vi "Operator Login Dialog.vi"(8 "error in (no error)":errorcluster, 9 "contextType":i32(ring) items=["Machine", "Domain", "ApplicationDirectory"]) -> (0 "error out":errorcluster, 1 "Groups":string[](array[string]), 2 "Operator Name":string, 3 "Logged In?":bool)   [LabVIEW 2020, in "Common Dialogs.lvlib"]
doc: "Use this template to create a dialog box with event handling."
uses:
  Common Dialogs.lvlib
  System.DirectoryServices.AccountManagement
panel:
  in  "Password":string
  in  "Operator Name":string
  in  "Cancel":bool
  in  "Login":bool
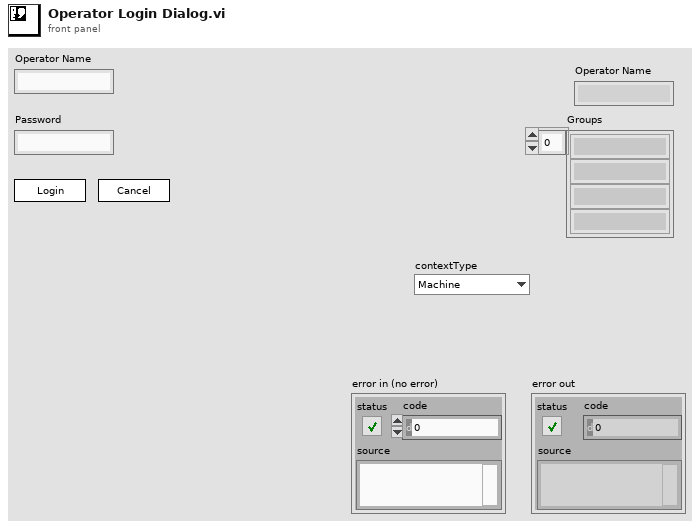
[diagram p1: front panel]
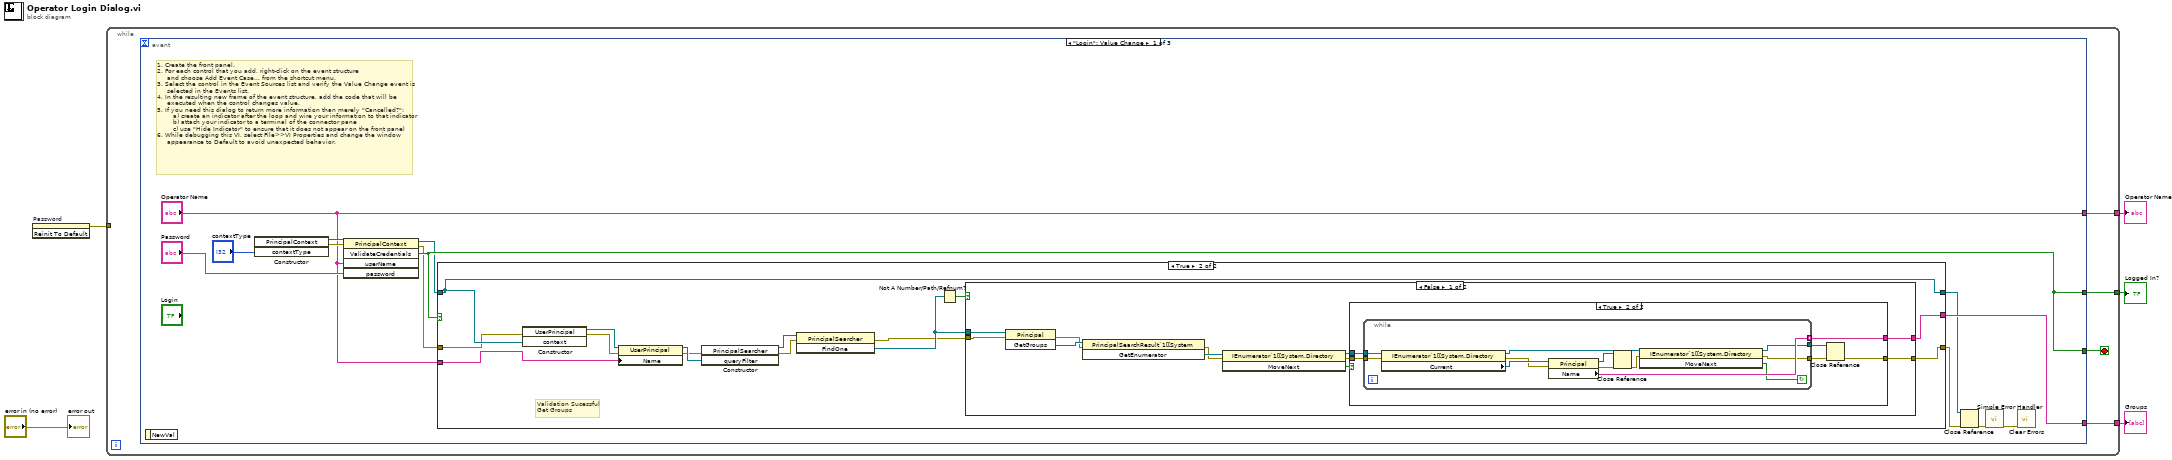
[diagram p0: block diagram]
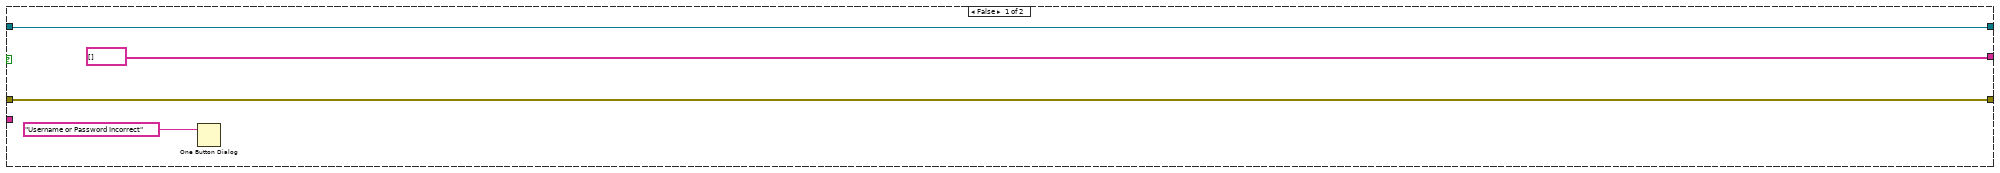
[diagram p2: hidden frame]
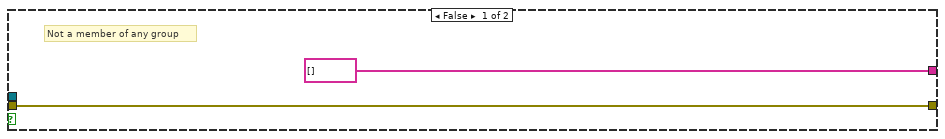
[diagram p3: hidden frame]
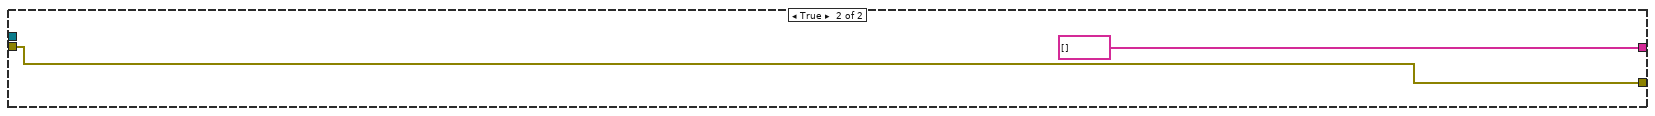
[diagram p4: hidden frame]
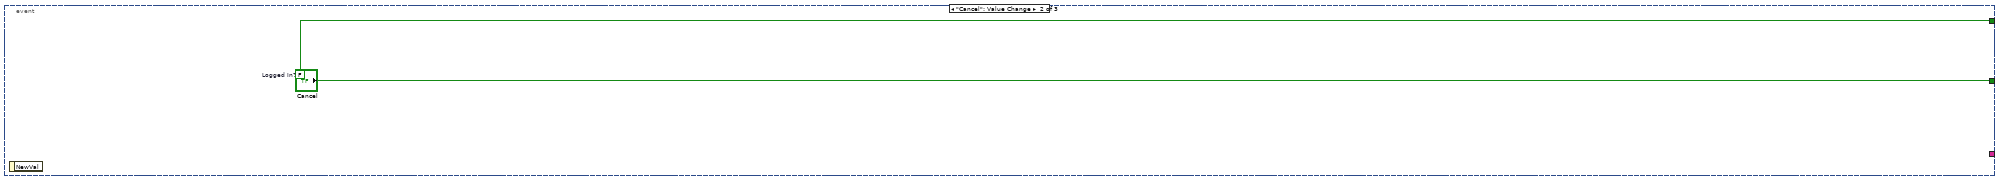
[diagram p5: hidden frame]
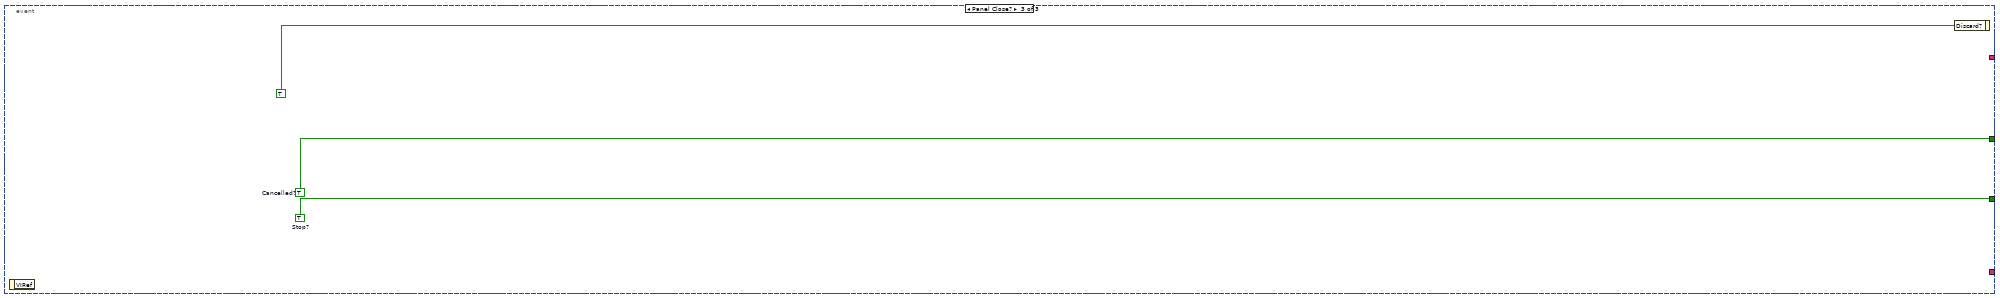
[diagram p6: hidden frame]
diagram:
  n1 = invoke on="Password" class="Str" method="Reinit To Default"() -> (error out=w2:errorcluster)  [unwired: 3 in, 2 out]
  n2 = while {
    tunnel: [w8] -> w5
    tunnel: [w7] -> w4
    tunnel: [w6] -> w3
    tunnel: w2 -> [_]
    stop <- w9 stop-if-true
    n3 = event shown="[0] \"Login\": Value Change" {
      selector: _ -> [_ _ _]
      dyn-events: _ -> [_ _ _]
      timeout: _ -> [_ _ _]
      tunnel: [w18 "Cancel" w77] -> w9
      tunnel: [w18 w75 w76] -> w8
      tunnel: ["Operator Name" _ _] -> w7
      tunnel: [w15 _ _] -> w6
      event "Login": Value Change {
        # "1. Create the front panel.\n2. For each control that you add, right-click on the event structure \n     and choose Add Event Case... from the shortcut menu.\n3. Select the control in the Event Sources list and verify the Value Change event is \n     selected in the Events list.\n4. In the resulting new frame of the event structure, add the code that will be \n     executed when the control changes value.\n5. If you need this dialog to return more information than merely \"Cancelled?\":\n        a) create an indicator after the loop and wire your information to that indicator\n        b) attach your indicator to a terminal of the connector pane\n        c) use \"Hide Indicator\" to ensure that it does not appear on the front panel\n6. While debugging this VI, select File>>VI Properties and change the window \n     appearance to Default to avoid unexpected behavior."
        n4 = event-data() -> ()  [unwired: 1 in, 1 out]
        n5 = constructor class="PrincipalContext"("contextType"="contextType") -> (reference out=w20:refnum<k24>, error out=w21:errorcluster)  [unwired: 3 in, 2 out]
        n6 = invoke class="PrincipalContext" method="ValidateCredentials"(reference=w20, error in=w21, "userName"="Operator Name", "password"="Password") -> (reference out=w14:refnum<k24>, error out=w13:errorcluster, "ValidateCredentials"=w18:bool)  [unwired: 1 in, 2 out]
        n7 = case shown="True" w18 {
          tunnel: [string[] [] ("Groups") w36] -> w15
          tunnel: w14 -> [w24 w40]
          tunnel: w13 -> [w25 w33]
          tunnel: [w25 w35] -> w12
          tunnel: [w24 w40] -> w11
          tunnel: "Operator Name" -> [_ w39]
          frame False {
            n8 = One Button Dialog(message="Username or Password Incorrect") -> ()  [unwired: 1 in, 1 out]
          }
          frame True {
            # "Validation Sucessful\nGet Groups"
            n9 = constructor class="UserPrincipal"(error in=w33, "context"=w40) -> (reference out=w32:refnum<k24>, error out=w31:errorcluster)  [unwired: 2 in, 2 out]
            n10 = property class="UserPrincipal"(reference=w32, error in=w31, "Name"=w39) -> (reference out=w30:refnum<k24>, error out=w29:errorcluster)
            n11 = constructor class="PrincipalSearcher"(error in=w29, "queryFilter"=w30) -> (reference out=w27:refnum<k24>, error out=w28:errorcluster)  [unwired: 2 in, 2 out]
            n12 = invoke class="PrincipalSearcher" method="FindOne"(reference=w27, error in=w28) -> (error out=w34:errorcluster, "FindOne"=w38:refnum<k24>)  [unwired: 1 in, 1 out]
            n13 = Not A Number/Path/Refnum?(number/path/refnum=w38) -> (NaN/Path/Refnum?=w37:bool)
            n14 = case shown="False" w37 {
              tunnel: w38 -> [w51 _]
              tunnel: [w45 string[] [] ("Groups")] -> w36
              tunnel: [w43 w73] -> w35
              tunnel: w34 -> [w42 w73]
              frame False {
                n15 = invoke class="Principal" method="GetGroups"(reference=w51, error in=w42) -> (error out=w41:errorcluster, "rvices.AccountManagement, Version=0.0.0.0, Culture=neutral, PublicKeyToken=b77a5c561934e089\tGetGroups"=w50:refnum<k24>)  [unwired: 1 in, 1 out]
                n16 = invoke class="PrincipalSearchResult`1[[System" method="GetEnumerator"(reference=w50, error in=w41) -> (error out=w48:errorcluster, "GetEnumerator"=w49:refnum<k24>)  [unwired: 1 in, 1 out]
                n17 = invoke class="IEnumerator`1[[System.Directory" method="MoveNext"(reference=w49, error in=w48) -> (reference out=w47:refnum<k24>, error out=w44:errorcluster, "MoveNext"=w46:bool)  [unwired: 1 in]
                n18 = case shown="True" w46 {
                  tunnel: w47 -> [_ w59]
                  tunnel: [string[] [] ("Groups") w57] -> w45
                  tunnel: w44 -> [w52 w58]
                  tunnel: [w52 w54] -> w43
                  frame False {
                    # "Not a member of any group"
                  }
                  frame True {
                    n19 = while {
                      tunnel: w59 -> [w71]
                      tunnel: w58 -> [w70]
                      tunnel: [w66] -> w57 mode=indexing
                      tunnel: [w64] -> w56
                      tunnel: [w60] -> w55
                      stop <- w65 continue-if-true
                      n20 = property class="IEnumerator`1[[System.Directory"(reference=w71, error in=w70) -> (reference out=w67:refnum<k24>, error out=w68:errorcluster, "Current"=w69:refnum<k24>)
                      n21 = property class="Principal"(reference=w69, error in=w68) -> (reference out=w63:refnum<k24>, error out=w62:errorcluster, "Name"=w66:string)
                      n22 = Close Reference(reference=w63, error in (no error)=w62) -> (error out=w61:errorcluster)
                      n23 = invoke class="IEnumerator`1[[System.Directory" method="MoveNext"(reference=w67, error in=w61) -> (reference out=w60:refnum<k24>, error out=w64:errorcluster, "MoveNext"=w65:bool)  [unwired: 1 in]
                    }
                    n24 = Close Reference(reference=w55, error in (no error)=w56) -> (error out=w54:errorcluster)
                  }
                }
              }
              frame True {
              }
            }
          }
        }
        n25 = Close Reference(reference=w11, error in (no error)=w12) -> (error out=w17:errorcluster)
        n26 = call <vilib>:"Simple Error Handler.vi"("error in (no error)"=w17) -> ("error out"=w16:errorcluster)  [unwired: 4 in, 4 out]
        n27 = call <vilib>:"Clear Errors.vi"("error in (no error)"=w16) -> ()  [unwired: 5 in, 2 out]
      }
      event "Cancel": Value Change {
        w75 = FALSE  # Logged In?
        n28 = event-data() -> ()  [unwired: 1 in, 1 out]
      }
      event Panel Close? {
        w76 = TRUE  # Cancelled?
        w77 = TRUE  # Stop?
        n29 = event-data() -> ()  [unwired: 1 in, 1 out]
        n30 = event-data("Discard?"=TRUE) -> ()  [unwired: 1 in, 1 out]
      }
    }
  }
  "Logged In?" <- w5
  "Operator Name" <- w4
  "Groups" <- w3
  "error out" <- "error in (no error)"
